vi "Set Memory Formatted.vi"(7 "Data":dbl[](array[numeric])=[0.0] format="%.2p", 8 "error in (no error)":errorcluster {"code" format="%.0x"}, 10 "Measurement":string, 11 "instrument handle":refnum<k15>) -> (0 "error out":errorcluster {"code" format="%.0x"}, 3 "instrument handle out":refnum<k15>)   [LabVIEW 2014, in "Agilent NA.lvlib"]
doc: "Set measurement data in the current format as set by the Measurement.Format property. Smith and Polar formats are not supported."
uses:
  Agilent NA.lvlib
  AgNA.dll
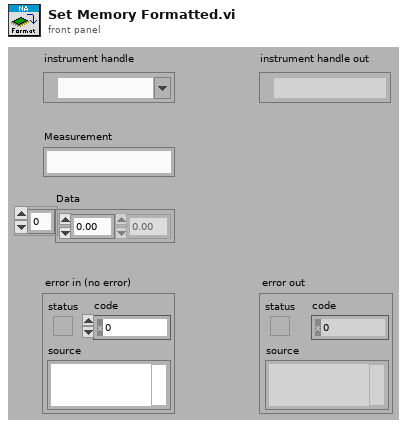
[diagram p1: front panel]
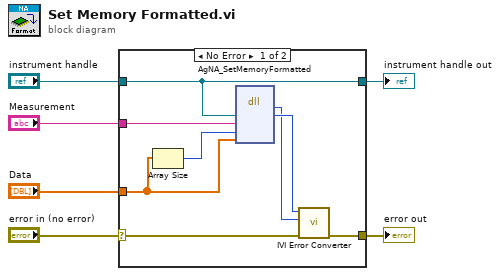
[diagram p0: block diagram]
diagram:
  n1 = case shown="No Error" "error in (no error)" {
    selector: "error in (no error)" -> [w12 w16]
    tunnel: [w11 w16] -> w6
    tunnel: "Measurement" -> [w10 _]
    tunnel: "Data" -> [w7 _]
    tunnel: [w9 w15] -> w2
    tunnel: "instrument handle" -> [w9 w15]
    frame No Error {
      n2 = Array Size(array=w7) -> (size(s)=w8:i32)
      n3 = dll-call lib="AgNA**.dll" fn="AgNA_SetMemoryFormatted"("Vi"=w9, "Measurement"=w10, "DataBufferSize"=w8, "Data"=w7) -> ("return type"=w13:i32, "Vi"=w14:u32)  [unwired: 6 in, 2 out]
      n4 = call "IVI Error Converter.vi"("error in (no error)"=w12, "IVI error code (0)"=w13, "instrument handle"=w14) -> ("error out"=w11:errorcluster)  [unwired: 7 in, 1 out]
    }
    frame Error {
    }
  }
  "error out" <- w6
  "instrument handle out" <- w2
